vi "Elapsed Timer.vi"(10 "Reset Timer":bool) -> (2 "Elapsed Time (ms)":u32)   [LabVIEW 2011]
panel:
  in  "Initial Tick Count":u32
  in  "Wrapped":bool
  in  "Previous Tick Count":u32
  # "Local Variables"
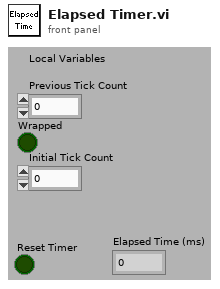
[diagram p1: front panel]
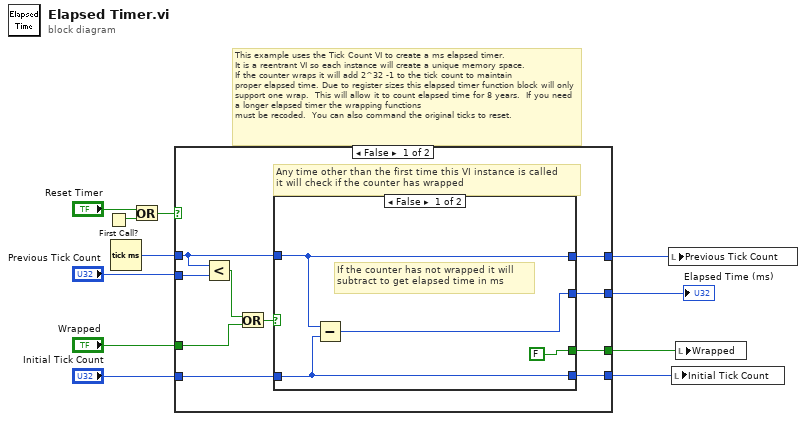
[diagram p0: block diagram]
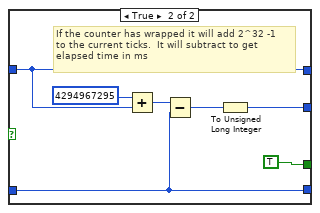
[diagram p2: hidden frame]
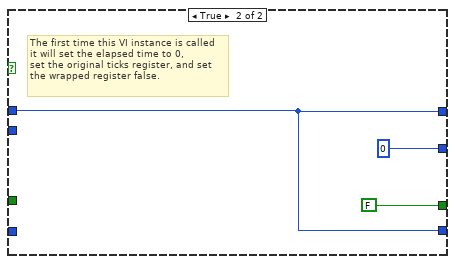
[diagram p3: hidden frame]
diagram:
  # "This example uses the Tick Count VI to create a ms elapsed timer.\nIt is a reentrant VI so each instance will create a unique memory space.\nIf the counter wraps it will add 2^32 -1 to the tick count to maintain\nproper elapsed time. Due to register sizes this elapsed timer function block will only support one wrap.  This will allow it to count elapsed time for 8 years.  If you need a longer elapsed timer the wrapping functions\nmust be recoded.  You can also command the original ticks to reset."
  n1 = First Call?() -> (First Call?: T/F=w1:bool)
  n2 = Tick Count (ms)() -> (millisecond timer value=w4:u32)
  n3 = Or(x="Reset Timer", y=w1) -> (x .or. y?=w3:bool)
  n4 = case shown="False" w3 {
    tunnel: [w20 u32 0] -> w5
    tunnel: [w21 w34] -> w6
    tunnel: "Initial Tick Count" -> [w19 _]
    tunnel: w4 -> [w17 w34]
    tunnel: [w18 w34] -> w8
    tunnel: "Previous Tick Count" -> [w16 _]
    tunnel: "Wrapped" -> [w13 _]
    tunnel: [w12 FALSE] -> w7
    frame False {
      # "Any time other than the first time this VI instance is called\nit will check if the counter has wrapped"
      n5 = Less?(x=w17, y=w16) -> (x < y?=w14:bool)
      n6 = Or(x=w14, y=w13) -> (x .or. y?=w15:bool)
      n7 = case shown="False" w15 {
        tunnel: w19 -> [w25 w32]
        tunnel: [w25 w32] -> w21
        tunnel: [w24 w28] -> w20
        tunnel: w17 -> [w22 w27]
        tunnel: [w22 w27] -> w18
        tunnel: [FALSE TRUE] -> w12
        frame False {
          # "If the counter has not wrapped it will \nsubtract to get elapsed time in ms"
          n8 = Subtract(x=w22, y=w25) -> (x-y=w24:u32)
        }
        frame True {
          # "If the counter has wrapped it will add 2^32 -1\nto the current ticks.  It will subtract to get \nelapsed time in ms"
          n9 = Add(x=u64 4294967295, y=w27) -> (x+y=w30:u64)
          n10 = Subtract(x=w30, y=w32) -> (x-y=w29:u64)
          n11 = To Unsigned Long Integer(number=w29) -> (unsigned 32bit integer=w28:u32)
        }
      }
    }
    frame True {
      # "The first time this VI instance is called\nit will set the elapsed time to 0, \nset the original ticks register, and set\nthe wrapped register false."
    }
  }
  "Elapsed Time (ms)" <- w5
  n12 = local write "Previous Tick Count"(w8) -> ()
  n13 = local write "Initial Tick Count"(w6) -> ()
  n14 = local write "Wrapped"(w7) -> ()
